vi "Get Number of Channels.vi"(4 "Pulsar Info":string) -> (1 "# Channels":i32)   [LabVIEW 2009]
uses:
  <vilib>/regexp/Match Regular Expression.xnode
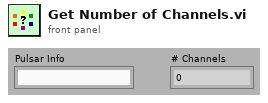
[diagram p1: front panel]
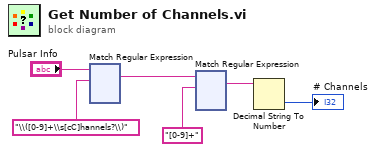
[diagram p0: block diagram]
diagram:
  n1 = xnode "Match Regular Expression"("input string"="Pulsar Info", "regular expression"="\\([0-9]+\\s[cC]hannels?\\)") -> ("whole match"=w3:string)  [unwired: 4 in, 4 out]
  n2 = xnode "Match Regular Expression"("input string"=w3, "regular expression"="[0-9]+") -> ("whole match"=w2:string)  [unwired: 4 in, 4 out]
  n3 = Decimal String To Number(string=w2) -> (number=→"# Channels":i32)  [unwired: 2 in, 1 out]
